vi "5.3.vi"() -> ()   [LabVIEW 2017]
panel:
  out "数组":i32[](array[numeric])
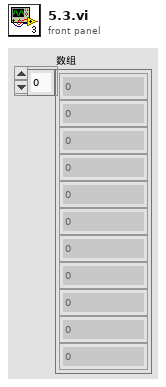
[diagram p1: front panel]
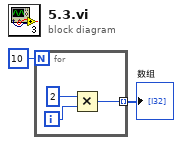
[diagram p0: block diagram]
diagram:
  n1 = for {
    N: 10 -> [_]
    tunnel: [w3] -> w1 mode=indexing
    i -> [w5]
    n2 = Multiply(x=2, y=w5) -> (x*y=w3:i32)
  }
  "数组" <- w1
